vi "Generate Error.vi"(8 "Error In":errorcluster, 10 "Error Type":T1) -> (0 "Error Out":errorcluster)   [LabVIEW 2011, in "LVH-LINX.lvlib"]
doc: "Generate a LINX error based on the Error Type input."
uses:
  LVH-LINX.lvlib
  Error Type.ctl
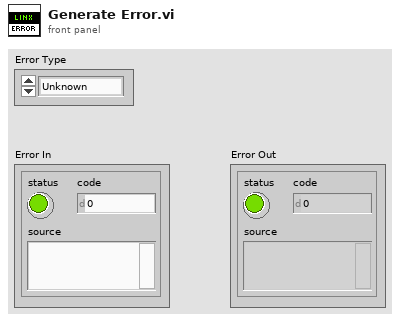
[diagram p1: front panel]
types:
  T1 = typedef "LVH-LINX.lvlib/Error Type.ctl" = enum16{"Unknown", "Timeout", "Corrupt Return Packet"}
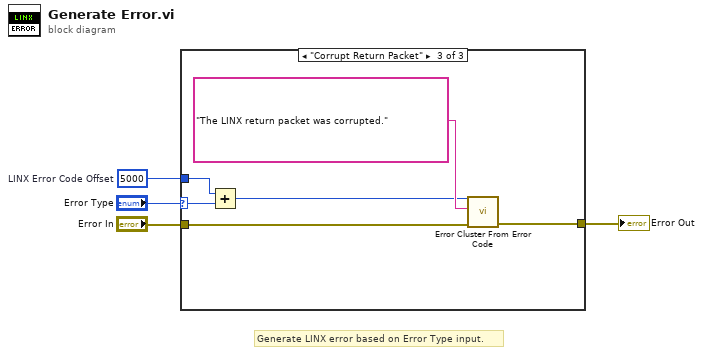
[diagram p0: block diagram]
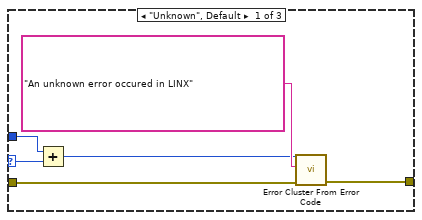
[diagram p2: hidden frame]
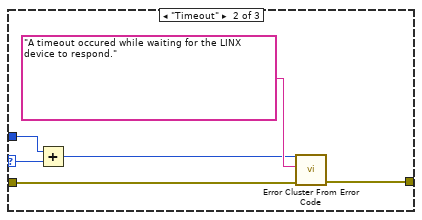
[diagram p3: hidden frame]
diagram:
  w2 = 5000  # LINX Error Code Offset
  # "Generate LINX error based on Error Type input."
  n1 = case shown="\"Corrupt Return Packet\"" "Error Type" {
    selector: "Error Type" -> [w6 w12 w18]
    tunnel: "Error In" -> [w9 w15 w21]
    tunnel: [w8 w14 w20] -> w3
    tunnel: w2 -> [w7 w13 w19]
    frame "Unknown", Default {
      n2 = Add(x=w7, y=w6) -> (x+y=w5:i32)
      n3 = call <vilib>:"Error Cluster From Error Code.vi"("error in (no error)"=w9, "error message (\"\")"="An unknown error occured in LINX" ("error message (\"\")"), "error code (0)"=w5) -> ("error out"=w8:errorcluster)  [unwired: 6 in]
    }
    frame "Timeout" {
      n4 = Add(x=w13, y=w12) -> (x+y=w11:i32)
      n5 = call <vilib>:"Error Cluster From Error Code.vi"("error in (no error)"=w15, "error message (\"\")"="A timeout occured while waiting for the LINX device to respond." ("error message (\"\")"), "error code (0)"=w11) -> ("error out"=w14:errorcluster)  [unwired: 6 in]
    }
    frame "Corrupt Return Packet" {
      n6 = Add(x=w19, y=w18) -> (x+y=w17:i32)
      n7 = call <vilib>:"Error Cluster From Error Code.vi"("error in (no error)"=w21, "error message (\"\")"="The LINX return packet was corrupted." ("error message (\"\")"), "error code (0)"=w17) -> ("error out"=w20:errorcluster)  [unwired: 6 in]
    }
  }
  "Error Out" <- w3
